vi "Resize Puzzle.vi"(11 "Puzzle Bounds":T1) -> (3 "picture":picture)   [LabVIEW 2021]
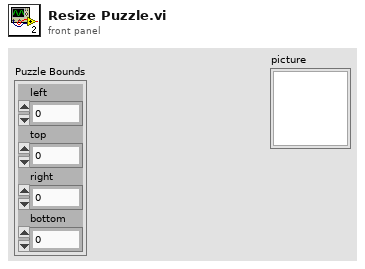
[diagram p1: front panel]
types:
  T1 = cluster{"left":i16, "top":i16, "right":i16, "bottom":i16}
  T2 = cluster{"Width":i16, "Style":enum32{"Solid", "Dash", "Dot", "DashDot", "DashDotDot"}}
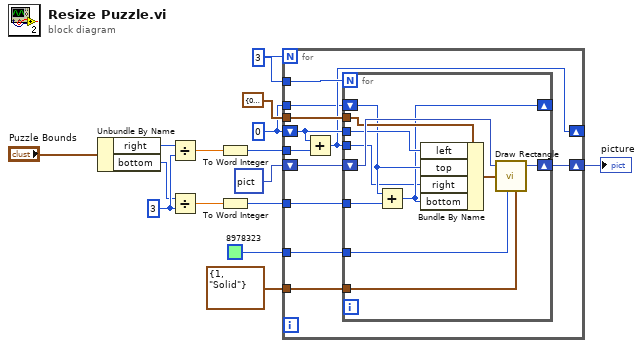
[diagram p0: block diagram]
diagram:
  w2 = i16 0 ("16bit integer")
  w13 = i16 3 ("y")
  w15 = 3
  n1 = Unbundle By Name("Puzzle Bounds") -> ("right"=w4:i16, "bottom"=w3:i16)
  n2 = Divide(x=w4, y=w13) -> (x/y=w10:dbl)
  n3 = Divide(x=w3, y=w13) -> (x/y=w8:dbl)
  n4 = To Word Integer(number=w10) -> (16bit integer=w9:i16)
  n5 = To Word Integer(number=w8) -> (16bit integer=w7:i16)
  n6 = for {
    N: w15 -> [_]
    tunnel: w15 -> [w26]
    shift-right: [w24] -> w5
    shift-left: picture data[5B] ("picture") -> [w25]
    shift-right: [w18] -> _
    shift-left: w2 -> [w23]
    tunnel: T1 {"left"=0, "top"=0, "right"=0, "bottom"=0} ("rect") -> [w22]
    tunnel: w9 -> [w19]
    tunnel: w7 -> [w21]
    tunnel: T2 {"Width"=1, "Style"=enum."Solid"} ("pen") -> [w20]
    tunnel: w2 -> [w17]
    tunnel: u32 8978323 ("color(black)") -> [w16]
    n7 = Add(x=w23, y=w19) -> (x+y=w18:i16)
    n8 = for {
      N: w26 -> [_]
      shift-right: [w36] -> w24
      shift-left: w25 -> [w37]
      shift-right: [w31] -> _
      shift-left: w17 -> [w32]
      tunnel: w22 -> [w34]
      tunnel: w21 -> [w35]
      tunnel: w20 -> [w29]
      tunnel: w18 -> [w28]
      tunnel: w23 -> [w33]
      tunnel: w16 -> [w27]
      n9 = Add(x=w32, y=w35) -> (x+y=w31:i16)
      n10 = Bundle By Name(cluster=w34, "left"=w33, "top"=w32, "right"=w28, "bottom"=w31) -> (w30:T1)
      n11 = call <vilib>:"Draw Rectangle.vi"("picture"=w37, "rect"=w30, "color(black)"=w27, "pen"=w29) -> ("new picture"=w36:picture)  [unwired: 5 in]
    }
  }
  "picture" <- w5
